vi "DeleteLayer.vi"(8 "error in":errorcluster, 11 "Icon.lvclass":refnum<class "Icon.lvclass">) -> (0 "error out":errorcluster, 3 "Icon.lvclass out":refnum<class "Icon.lvclass">)   [LabVIEW 2020, in "Icon.lvclass"]
doc: "Delete an existing User Layer"
uses:
  Icon.lvclass
  Icon.lvclass/Icon.ctl
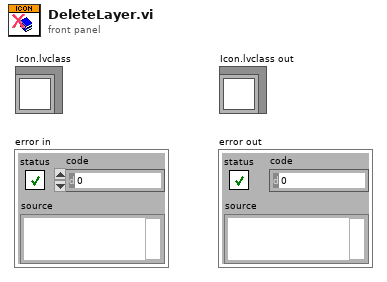
[diagram p1: front panel]
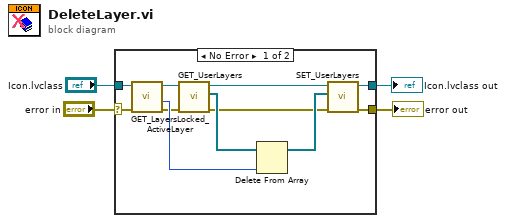
[diagram p0: block diagram]
diagram:
  n1 = case shown="No Error" "error in" {
    selector: "error in" -> [w5 w16]
    tunnel: [w12 w16] -> w4
    tunnel: [w10 w17] -> w3
    tunnel: "Icon.lvclass" -> [w6 w17]
    frame No Error {
      n2 = call-dynamic "GET_LayersLocked_ActiveLayer.vi"("error in (no error)"=w5, "Icon.lvclass in"=w6) -> ("error out"=w8:errorcluster, "Active Layer"=w15:i32, "Icon.lvclass out"=w7:refnum<class "Icon.lvclass">)  [unwired: 7 out]
      n3 = call-dynamic "GET_UserLayers.vi"("error in (no error)"=w8, "Icon.lvclass in"=w7) -> ("error out"=w11:errorcluster, "All Layers"=w13:refnum<class "Layer.lvclass">[], "Icon.lvclass out"=w9:refnum<class "Icon.lvclass">)  [unwired: 7 out]
      n4 = Delete From Array(array=w13, index=w15) -> (array with subset deleted=w14:refnum<class "Layer.lvclass">[])  [unwired: 1 in, 1 out]
      n5 = call-dynamic "SET_UserLayers.vi"("error in (no error)"=w11, "Layers"=w14, "Icon.lvclass in"=w9) -> ("error out"=w12:errorcluster, "Icon.lvclass out"=w10:refnum<class "Icon.lvclass">)  [unwired: 7 out]
    }
    frame Error {
    }
  }
  "error out" <- w4
  "Icon.lvclass out" <- w3
